vi "I2C_EXP_Port.vi"(6 "LINX Resource in":T1, 7 "EXP1_Port 1":bool[](array[boolean]), 8 "error in (no error)":errorcluster, 9 "I2C_Channel_platform":T7, 10 "I2C Slave Address (0)":u8=116 format="%.0x", 11 "EXP1_Port0":bool[](array[boolean])) -> (0 "error out":errorcluster, 2 "appended array":u8[](array[numeric]), 3 "LINX Resource out":T1)   [LabVIEW 2014]
uses:
  <vilib>/MakerHub/LINX/Private/Type Defs/LINX Ref.ctl
  <vilib>/MakerHub/LINX/Private/Type Defs/Platform.ctl
  <vilib>/MakerHub/LINX/Private/Type Defs/Interface.ctl
  <vilib>/MakerHub/LINX/Private/Device/Type Defs/LINX Device Config.ctl
  <vilib>/MakerHub/LINX/Private/Device/Type Defs/TCP Config.ctl
  <vilib>/MakerHub/LINX/Private/Device/Type Defs/Channels.ctl
  User Defined/I2C_Platform_Selector.ctl
  <vilib>/MakerHub/LINX/Private/Type Defs/Peripherals/I2C/EOF.ctl
  <vilib>/MakerHub/LINX/Private/Local IO/LinxI2cWrite.vi
  <vilib>/MakerHub/LINX/Public/Utilities/Check Channel.vi
  <vilib>/MakerHub/LINX/Private/Local IO/Handle Errors.vi
  <vilib>/MakerHub/LINX/Private/Utilties/Generate Error.vi
  <vilib>/MakerHub/LINX/LMH-LINX.lvlib
  <vilib>/MakerHub/LINX/Private/Device/Device.lvlib
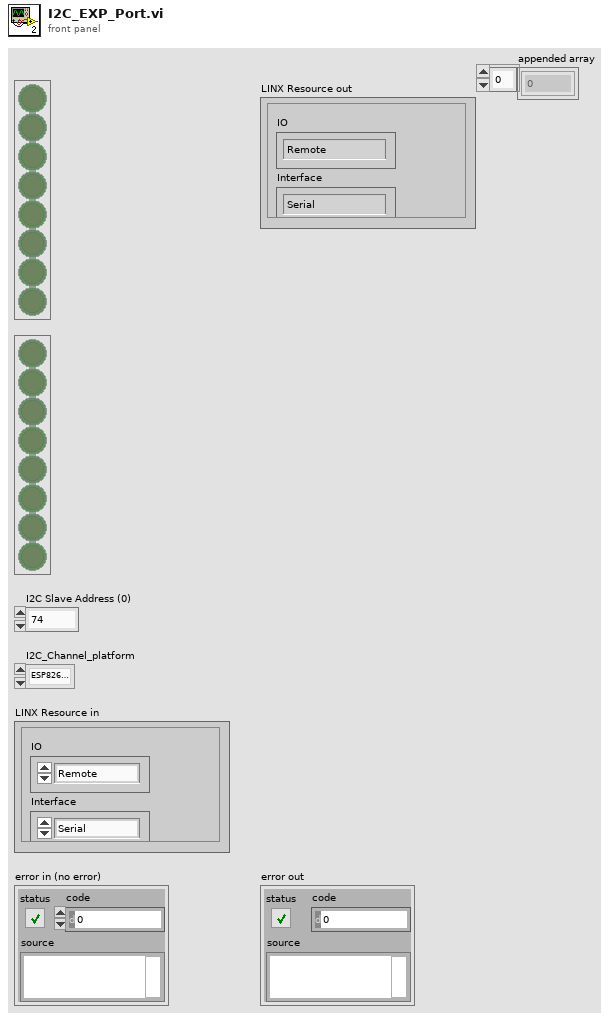
[diagram p1: front panel]
types:
  T1 = typedef "LMH-LINX.lvlib/LINX Ref.ctl" = cluster{"IO":T2, "Interface":T3, "LINX Device Config":T4}
  T2 = typedef "LMH-LINX.lvlib/Platform.ctl" = enum16{"Remote", "Local"}
  T3 = typedef "LMH-LINX.lvlib/Interface.ctl" = enum16{"Serial", "TCP"}
  T4 = typedef "LMH-LINX.lvlib/Device.lvlib/LINX Device Config.ctl" = cluster{"Interface":T3, "COM Port":refnum<visa-resource-name>, "TCP Configuration":T5, "Device Family":u8, "Device ID":u8, "Device Name":string, "TCP Ref":refnum<k5>, "Channels":T6}
  T5 = typedef "LMH-LINX.lvlib/Device.lvlib/TCP Config.ctl" = cluster{"IP Address":string, "Port":u16}
  T6 = typedef "LMH-LINX.lvlib/Channels.ctl" = cluster{"DI":u8[], "DO":u8[], "AI":u8[], "AO":u8[], "PWM":u8[], "QE":u8[], "UART":u8[], "I2C 2":u8[], "SPI":u8[], "CAN":u8[], "Servo":u8[], "AI Ref (V)":dbl, "AI Resolution (Bits)":u8, "AO Ref (V)":dbl, "AO Resolution (Bits)":u8}
  T7 = typedef "I2C_Platform_Selector.ctl" = enum16{"ESP8266-I2C", "Raspberry Pi-I2C"}
  T8 = typedef "LMH-LINX.lvlib/EOF.ctl" = enum8{"Stop", "Restart", "Restart No Stop", "No Stop"}
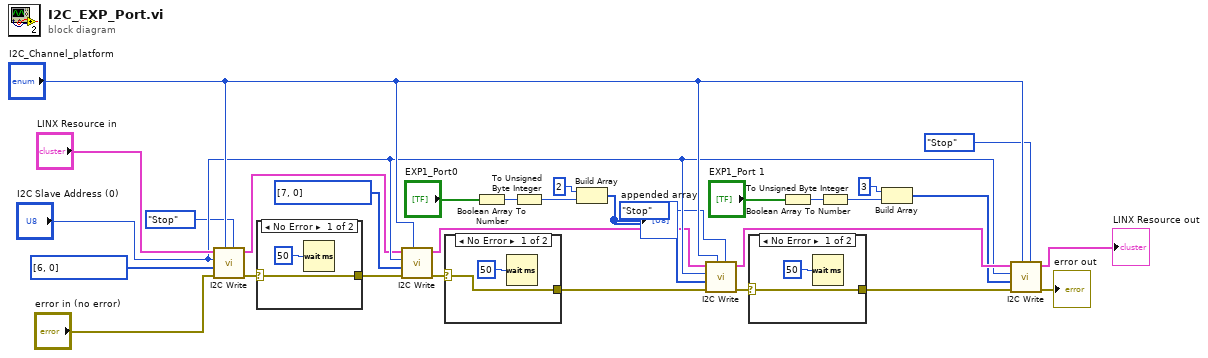
[diagram p0: block diagram]
diagram:
  n1 = call <vilib>:"I2C Write.vi"("EOF"=EOF."Stop", "I2C Channel"="I2C_Channel_platform", "Error In"="error in (no error)", "Data"=u8[] [6, 0], "I2C Slave Address (0)"="I2C Slave Address (0)", "LINX Resource"="LINX Resource in") -> ("Error Out"=w2:errorcluster, "LINX Resource"=w7:T1)  [unwired: 4 in]
  n2 = case shown="No Error" w2 {
    selector: w2 -> [w31 w33]
    tunnel: [w31 w33] -> w8
    frame No Error {
      n3 = Wait (ms)(milliseconds to wait=u32 50) -> ()  [unwired: 1 out]
    }
    frame Error {
    }
  }
  n4 = call <vilib>:"I2C Write.vi"("I2C Channel"="I2C_Channel_platform", "Error In"=w8, "Data"=u8[] [7, 0], "I2C Slave Address (0)"="I2C Slave Address (0)", "LINX Resource"=w7) -> ("Error Out"=w9:errorcluster, "LINX Resource"=w6:T1)  [unwired: 5 in]
  n5 = case shown="No Error" w9 {
    selector: w9 -> [w34 w36]
    tunnel: [w34 w36] -> w10
    frame No Error {
      n6 = Wait (ms)(milliseconds to wait=u32 50) -> ()  [unwired: 1 out]
    }
    frame Error {
    }
  }
  n7 = Boolean Array To Number(Boolean array="EXP1_Port0") -> (number=w16:u32)
  n8 = To Unsigned Byte Integer(number=w16) -> (unsigned 8bit integer=w17:u8)
  n9 = Build Array(u8 2 ("I2C Slave Address 2"), w17) -> (w18:u8[])
  "appended array" <- w18
  n10 = call <vilib>:"I2C Write.vi"("EOF"=EOF."Stop", "I2C Channel"="I2C_Channel_platform", "Error In"=w10, "Data"=w18, "I2C Slave Address (0)"="I2C Slave Address (0)", "LINX Resource"=w6) -> ("Error Out"=w14:errorcluster, "LINX Resource"=w28:T1)  [unwired: 4 in]
  n11 = case shown="No Error" w14 {
    selector: w14 -> [w38 _]
    tunnel: [w38 _] -> w27
    frame No Error {
      n12 = Wait (ms)(milliseconds to wait=u32 50) -> ()  [unwired: 1 out]
    }
    frame Error {
    }
  }
  n13 = Boolean Array To Number(Boolean array="EXP1_Port 1") -> (number=w20:u32)
  n14 = To Unsigned Byte Integer(number=w20) -> (unsigned 8bit integer=w19:u8)
  n15 = Build Array(u8 3 ("I2C Slave Address 2"), w19) -> (w22:u8[])
  n16 = call <vilib>:"I2C Write.vi"("EOF"=EOF."Stop", "I2C Channel"="I2C_Channel_platform", "Error In"=w27, "Data"=w22, "I2C Slave Address (0)"="I2C Slave Address (0)", "LINX Resource"=w28) -> ("Error Out"=→"error out":errorcluster, "LINX Resource"=→"LINX Resource out":T1)  [unwired: 4 in]
